vi "Untitled 6 (SubVI).vi"() -> (0 "error out":errorcluster, 1 "READ LSB CAL_PARAM 2":u8[][](array[numeric]) format="%.0x", 2 "Array 3":i16[][](array[numeric]), 3 "Device_ID 2":u8[](array[numeric]) format="%.0x", 4 "Array":u16[][](array[numeric]), 5 "READ MSB CAL_PARAM 2":u8[][](array[numeric]) format="%.0x")   [LabVIEW 2016]
uses:
  <vilib>/myRIO/Instrument Drivers/Onboard IO/I2C/typedefs/I2C User Configuration.ctl
  <vilib>/myRIO/Instrument Drivers/Onboard IO/I2C/typedefs/I2C Transfer Rate.ctl
  <vilib>/myRIO/Instrument Drivers/Onboard IO/I2C/typedefs/I2C Reference.ctl
  <vilib>/myRIO/Common/Instrument Driver Framework/Utilities/typedefs/myRIO Generic Hardware Reference.ctl
  <vilib>/myRIO/Common/Instrument Driver Framework/Utilities/typedefs/Hardware Version Enum.ctl
  <vilib>/myRIO/Common/Instrument Driver Framework/Utilities/typedefs/myRIO v1.0 Reference.ctl
  <vilib>/myRIO/Common/Instrument Driver Framework/Utilities/typedefs/Generic FPGA Reference.ctl
  <vilib>/myRIO/Common/Instrument Driver Framework/myRIO v1.0/I2C/typedefs/I2C Channels Enum.ctl
  <vilib>/myRIO/Instrument Drivers/Onboard IO/I2C/typedefs/I2C Configuration.ctl
  <vilib>/userdefined/High Color/nirio_resource_hc.ctl
  <vilib>/myRIO/Common/Instrument Driver Framework/Utilities/vis/Is FPGA Ref Available.vi
  <vilib>/myRIO/Common/Instrument Driver Framework/myRIO v1.0/I2C/vis/myRIO v1.1 Open I2C.vi
  <vilib>/myRIO/Instrument Drivers/Onboard IO/I2C/vis/Configure.vi
  <vilib>/myRIO/Instrument Drivers/Onboard IO/I2C/vis/Write Read.vi
  <vilib>/myRIO/Common/Instrument Driver Framework/Utilities/vis/Validate Channels.vi
  <vilib>/myRIO/Common/Instrument Driver Framework/myRIO v1.0/I2C/vis/myRIO v1.0 Reserve I2C.vi
  <vilib>/myRIO/Common/Instrument Driver Framework/myRIO v1.0/I2C/vis/myRIO v1.0 Build MUX Configuration I2C.vi
  <vilib>/myRIO/Common/Instrument Driver Framework/myRIO v1.0/Resource Manager/vis/myRIO v1.0 Reserve Channel List.vi
  <vilib>/myRIO/Common/Instrument Driver Framework/myRIO v1.0/Resource Manager/vis/myRIO v1.0 Create Configuration List.vi
  <vilib>/myRIO/Common/Instrument Driver Framework/myRIO v1.0/Resource Manager/vis/myRIO v1.0 Reserve Channel.vi
  <vilib>/myRIO/Common/Instrument Driver Framework/myRIO v1.0/Resource Manager/vis/myRIO v1.0 Unreserve Channel.vi
  <vilib>/myRIO/Common/Instrument Driver Framework/myRIO v1.0/Resource Manager/vis/myRIO v1.0 Build Mutex Name.vi
  <vilib>/Utility/VariantDataType/GetNumericInfo.vi
  <vilib>/Utility/error.llb/Error Cluster From Error Code.vi
  <vilib>/myRIO/Common/Instrument Driver Framework/myRIO v1.0/myRIO v1.1 Open.vi
  <vilib>/myRIO/Common/Instrument Driver Framework/Utilities/vis/IO Manager.vi
  <vilib>/myRIO/Common/Instrument Driver Framework/Utilities/vis/Configuration Manager.vi
  <vilib>/myRIO/Common/Instrument Driver Framework/myRIO v1.0/Resource Manager/vis/myRIO v1.0 Configure IO.vi
  <vilib>/myRIO/Common/Instrument Driver Framework/myRIO v1.0/myRIO v1.0 Close.vi
  <vilib>/myRIO/Common/Instrument Driver Framework/myRIO v1.0/I2C/vis/myRIO v1.0 Configure I2C.vi
  <vilib>/myRIO/Common/Instrument Driver Framework/myRIO v1.0/I2C/vis/myRIO v1.0 Write I2C.vi
  <vilib>/myRIO/Common/Instrument Driver Framework/myRIO v1.0/I2C/vis/myRIO v1.0 Read I2C.vi
  <vilib>/myRIO/Express VI/Onboard IO/I2C/I2C Express VI.xnode
  <vilib>/myRIO/Instrument Drivers/Onboard IO/I2C/vis/myRIO I2C Open.xnode
  <vilib>/myRIO/Instrument Drivers/Onboard IO/I2C/I2C.lvlib
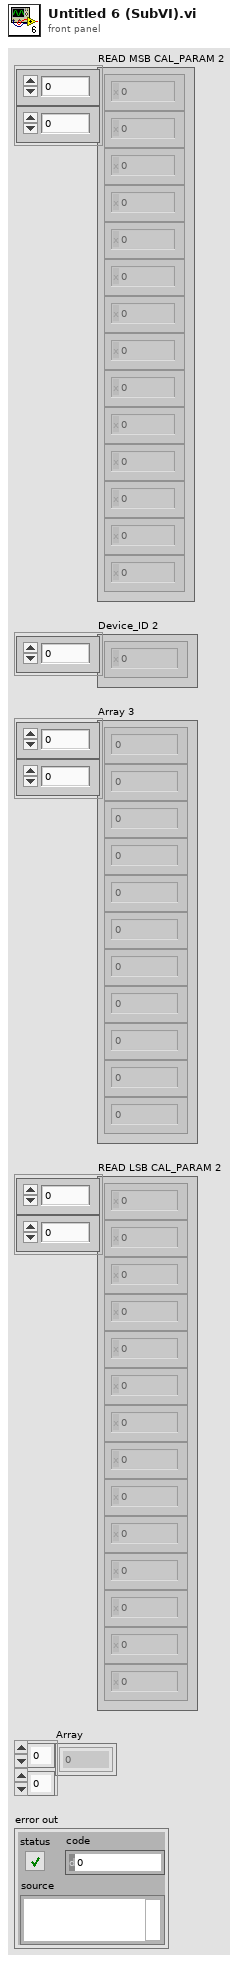
[diagram p1: front panel]
types:
  T1 = typedef "I2C.lvlib/I2C Reference.ctl" = cluster{"myRIO Reference":T2, "I2C Channels Enum":T6, "I2C Configuration":T7}
  T2 = typedef "myRIO Generic Hardware Reference.ctl" = cluster{"myRIO Model":T3, "myRIO Hardware Reference":T4}
  T3 = typedef "Hardware Version Enum.ctl" = enum16{"Unknown", "myRIO-1900", "myRIO-1950", "roboRIO", "NI ELVIS RIO CM"}
  T4 = typedef "myRIO v1.0 Reference.ctl" = cluster{"Generic FPGA Reference":T5, "Allow multiple opens":bool}
  T5 = typedef "Generic FPGA Reference.ctl" = refnum<k20>
  T6 = typedef "I2C Channels Enum.ctl" = enum16{"Not Connected", "A/I2C", "B/I2C", "I2C/I2C"}
  T7 = typedef "I2C.lvlib/I2C Configuration.ctl" = cluster{"I2C Transfer Rate":T8}
  T8 = typedef "I2C.lvlib/I2C Transfer Rate.ctl" = enum16{"Standard mode (100 kbps)", "Fast mode (400 kbps)"}
  T9 = typedef "I2C.lvlib/I2C User Configuration.ctl" = cluster{"I2C Transfer Rate":T8}
  T10 = typedef "nirio_resource_hc.ctl" = tag
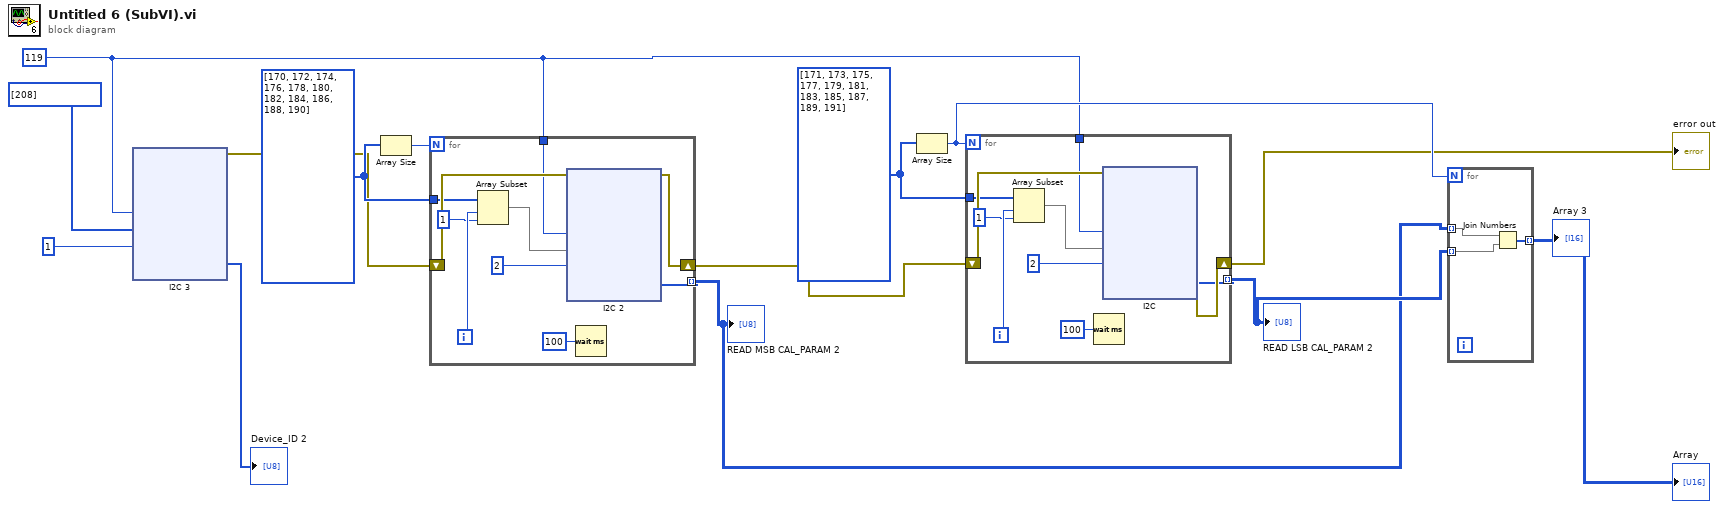
[diagram p0: block diagram]
diagram:
  w7 = u8[] [171, 173, 175, 177, 179, 181, 183, 185, 187, 189, 191] ("Slave Address (7-bit)")
  w6 = u8[] [170, 172, 174, 176, 178, 180, 182, 184, 186, 188, 190] ("Slave Address (7-bit)")
  w8 = u8 119 ("Slave Address (7-bit)")
  n1 = xnode "I2C 3"("Slave Address (7-bit)"=w8, "Bytes to Write"=u8[] [208] ("Slave Address (7-bit)"), "Byte Count"=u32 1) -> ("Bytes Read"=→"Device_ID 2":u8[], "error out"=w4:errorcluster)  [unwired: 1 in]
  n2 = Array Size(array=w6) -> (size(s)=w5:i32)
  n3 = for {
    N: w5 -> [_]
    tunnel: w8 -> [w22]
    shift-right: [w23] -> w9
    shift-left: w4 -> [w24]
    tunnel: [w21] -> w12 mode=indexing
    tunnel: w6 -> [w19]
    i -> [w17]
    n4 = Array Subset(array=w19, index=w17, length=1 ("Länge")) -> (w18:u8[])
    n5 = xnode "I2C 2"("Slave Address (7-bit)"=w22, "Bytes to Write"=w18, "Byte Count"=u32 2, "error in (no error)"=w24) -> ("Bytes Read"=w21:u8[], "error out"=w23:errorcluster)
    n6 = Wait (ms)(milliseconds to wait=u32 100 ("Zu wartende ms")) -> ()  [unwired: 1 out]
  }
  "READ MSB CAL_PARAM 2" <- w12
  n7 = Array Size(array=w7) -> (size(s)=w11:i32)
  n8 = for {
    N: w11 -> [_]
    tunnel: w8 -> [w72]
    shift-right: [w73] -> w10
    shift-left: w9 -> [w74]
    tunnel: [w71] -> w13 mode=indexing
    tunnel: w7 -> [w69]
    i -> [w67]
    n9 = Array Subset(array=w69, index=w67, length=1 ("Länge")) -> (w68:u8[])
    n10 = Wait (ms)(milliseconds to wait=u32 100 ("Zu wartende ms")) -> ()  [unwired: 1 out]
    n11 = xnode "I2C"("Slave Address (7-bit)"=w72, "Bytes to Write"=w68, "Byte Count"=u32 2, "error in (no error)"=w74) -> ("Bytes Read"=w71:u8[], "error out"=w73:errorcluster)
  }
  "READ LSB CAL_PARAM 2" <- w13
  "error out" <- w10
  n12 = for {
    N: w11 -> [_]
    tunnel: w12 -> [w117] mode=indexing
    tunnel: w13 -> [w116] mode=indexing
    tunnel: [w115] -> w14 mode=indexing
    n13 = Join Numbers(hi=w117, lo=w116) -> ((hi.lo)=w115:u16[])
  }
  "Array 3" <- w14
  "Array" <- w14
